vi "niRFUtil FWK Get Instrument Version Info.vi"(9 "error in (no error)":errorcluster, 10 "Class Name":string) -> (1 "error out":errorcluster, 2 "Instr Info":T1={"Check Version?"=TRUE, "Instr type"=enum."RFInstr Agn", "Major Version"="1", "Minor Version"="1", "Registry Key"=[], "Product Name"="NI"})   [LabVIEW 2015, in "niRFUtil.lvlib"]
uses:
  niRFUtil.lvlib
  Includes/niRFUtil INC FWK Instrument Version Info.ctl
  Includes/niRFUtil INC FWK Class Types.ctl
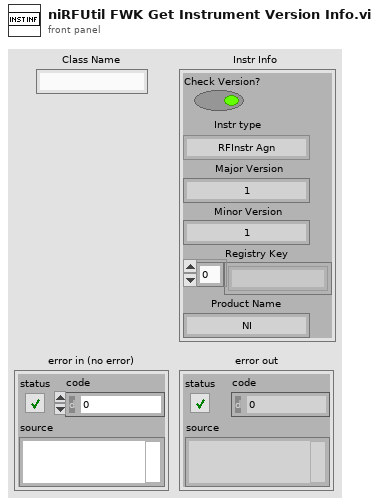
[diagram p1: front panel]
types:
  T1 = typedef "niRFUtil.lvlib/niRFUtil INC FWK Instrument Version Info.ctl" = cluster{"Check Version?":bool, "Instr type":T2, "Major Version":string, "Minor Version":string, "Registry Key":string[], "Product Name":string}
  T2 = typedef "niRFUtil.lvlib/niRFUtil INC FWK Class Types.ctl" = enum16{"RFInstr Agn", "RFSAInstr", "DCPowerInstr"}
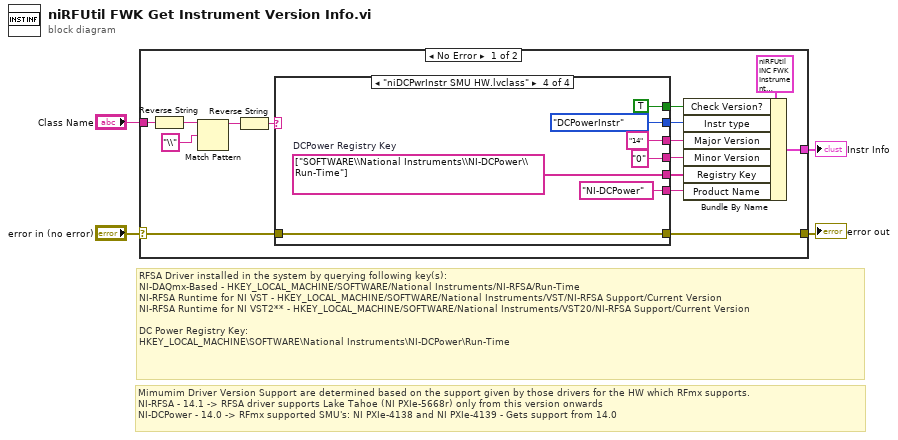
[diagram p0: block diagram]
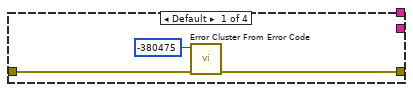
[diagram p2: hidden frame]
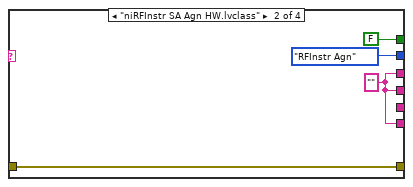
[diagram p3: hidden frame]
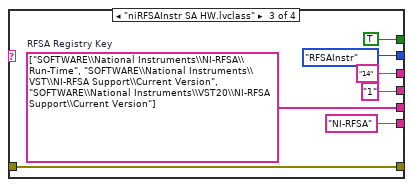
[diagram p4: hidden frame]
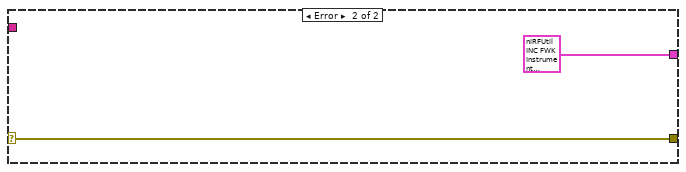
[diagram p5: hidden frame]
diagram:
  # "Mimumim Driver Version Support are determined based on the support given by those drivers for the HW which RFmx supports.\nNI-RFSA - 14.1 -> RFSA driver supports Lake Tahoe (NI PXIe-5668r) only from this version onwards\nNI-DCPower - 14.0 -> RFmx supported SMU's: NI PXIe-4138 and NI PXIe-4139 - Gets support from 14.0"
  # "RFSA Driver installed in the system by querying following key(s):\nNI-DAQmx-Based - HKEY_LOCAL_MACHINE/SOFTWARE/National Instruments/NI-RFSA/Run-Time\nNI-RFSA Runtime for NI VST - HKEY_LOCAL_MACHINE/SOFTWARE/National Instruments/VST/NI-RFSA Support/Current Version\nNI-RFSA Runtime for NI VST2** - HKEY_LOCAL_MACHINE/SOFTWARE/National Instruments/VST20/NI-RFSA Support/Current Version\n\nDC Power Registry Key:\nHKEY_LOCAL_MACHINE\\SOFTWARE\\National Instruments\\NI-DCPower\\Run-Time"
  n1 = case shown="No Error" "error in (no error)" {
    selector: "error in (no error)" -> [w6 w42]
    tunnel: [w19 T1 {"Check Version?"=FALSE, "Instr type"=enum."RFInstr Agn", "Major Version"="0", "Minor Version"="0", "Registry Key"=[], "Product Name"=""} ("Instr Info 2")] -> w4
    tunnel: [w5 w42] -> w2
    tunnel: "Class Name" -> [w10 _]
    frame No Error {
      n2 = Reverse String(1:w10) -> (0:w11:string)
      n3 = Match Pattern(string=w11, regular expression="\\") -> (before substring=w13:string)  [unwired: 1 in, 3 out]
      n4 = Reverse String(1:w13) -> (0:w9:string)
      n5 = case shown="\"niDCPwrInstr SMU HW.lvclass\"" w9 {
        tunnel: [_ FALSE TRUE TRUE] -> w17
        tunnel: [_ niRFUtil_INC_FWK_Class_Types."RFInstr Agn" ("Instr type") niRFUtil_INC_FWK_Class_Types."RFSAInstr" ("Instr type") niRFUtil_INC_FWK_Class_Types."DCPowerInstr" ("Instr type")] -> w16
        tunnel: [_ w24 "14" "14"] -> w15
        tunnel: [_ w24 "1" "0"] -> w14
        tunnel: [_ _ w29 w36] -> w8
        tunnel: [_ w24 "NI-RFSA" "NI-DCPower"] -> w7
        tunnel: w6 -> [w22 w23 w27 w34]
        tunnel: [w21 w23 w27 w34] -> w5
        frame Default {
          n6 = call <vilib>:"Error Cluster From Error Code.vi"("error in (no error)"=w22, "error code (0)"=-380475) -> ("error out"=w21:errorcluster)  [unwired: 7 in]
        }
        frame "niRFInstr SA Agn HW.lvclass" {
          w24 = ""
        }
        frame "niRFSAInstr SA HW.lvclass" {
          w29 = string[] ["SOFTWARE\\National Instruments\\NI-RFSA\\Run-Time", "SOFTWARE\\National Instruments\\VST\\NI-RFSA Support\\Current Version", "SOFTWARE\\National Instruments\\VST20\\NI-RFSA Support\\Current Version"]  # RFSA Registry Key
        }
        frame "niDCPwrInstr SMU HW.lvclass" {
          w36 = string[] ["SOFTWARE\\National Instruments\\NI-DCPower\\Run-Time"]  # DCPower Registry Key
        }
      }
      n7 = Bundle By Name(cluster=T1 {"Check Version?"=FALSE, "Instr type"=enum."RFInstr Agn", "Major Version"="0", "Minor Version"="0", "Registry Key"=[], "Product Name"=""} ("Instr Info 2"), "Check Version?"=w17, "Instr type"=w16, "Major Version"=w15, "Minor Version"=w14, "Registry Key"=w8, "Product Name"=w7) -> (w19:T1)
    }
    frame Error {
    }
  }
  "Instr Info" <- w4
  "error out" <- w2
